vi "枚举全局.vi"() -> ()   [LabVIEW 2014]
panel:
  out "枚举":T1(ring)
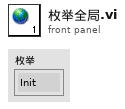
[diagram p1: front panel]
types:
  T1 = enum16{"Init", "Loop", "Write LOFF", "Write LON", "Read", "Exit", "Open", "Close"}
diagram:
